vi "Read PageSelector Visible.vi"(9 "PageSelector in":refnum<class "PageSelector.lvclass">) -> (3 "PageSelector out":refnum<class "PageSelector.lvclass">, 4 "Visible":bool)   [LabVIEW 2014, in "Raspberry Pi Compatible Compiler for LabVIEW.lvlib" / "PageSelector.lvclass"]
uses:
  PageSelector.lvclass
  PageSelector.lvclass/PageSelector.ctl
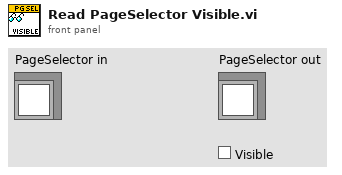
[diagram p1: front panel]
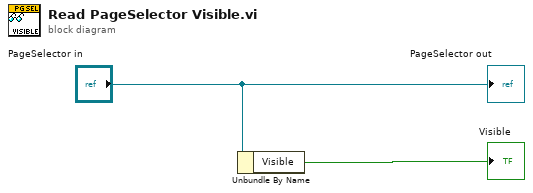
[diagram p0: block diagram]
diagram:
  n1 = Unbundle By Name("PageSelector in") -> ("Visible"=→"Visible":bool)
  "PageSelector out" <- "PageSelector in"
